vi "Write Roles.vi"(8 "error in (no error)":errorcluster, 10 "Roles":T1, 11 "PreparePassInGame1 in":refnum<class "PreparePassInGame1.lvclass">) -> (0 "error out":errorcluster, 3 "PreparePassInGame1 out":refnum<class "PreparePassInGame1.lvclass">)   [LabVIEW 2020, in "PreparePassInGame1.lvclass"]
uses:
  PreparePassInGame1.lvclass
  ShootRole_class/ShootRole.lvclass
  PreparePassReceiverRole_class/PreparePassReceiverRole.lvclass
  PreparePassInGame1.lvclass/PreparePassInGame1.ctl
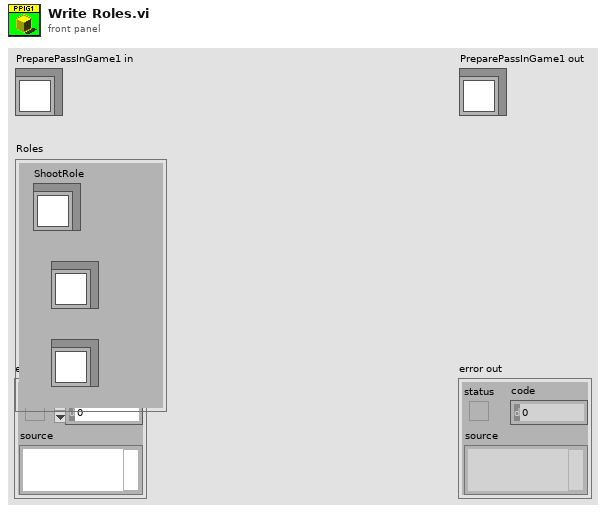
[diagram p1: front panel]
types:
  T1 = cluster{"ShootRole":refnum<class "ShootRole.lvclass">, "PreparePassReceiverRole1":refnum<class "PreparePassReceiverRole.lvclass">, "PreparePassReceiverRole2":refnum<class "PreparePassReceiverRole.lvclass">}
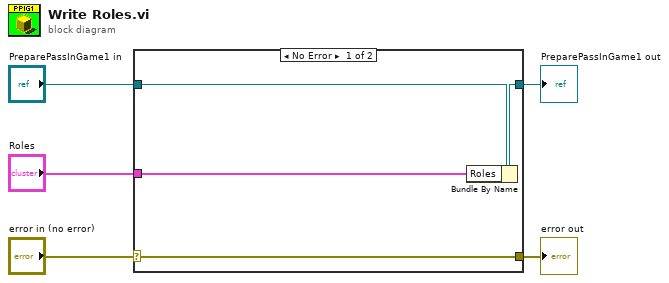
[diagram p0: block diagram]
diagram:
  n1 = case shown="No Error" "error in (no error)" {
    selector: "error in (no error)" -> [w9 w10]
    tunnel: [w9 w10] -> w4
    tunnel: [w7 w11] -> w2
    tunnel: "PreparePassInGame1 in" -> [w8 w11]
    tunnel: "Roles" -> [w6 _]
    frame No Error {
      n2 = Bundle By Name(cluster=w8, "Roles"=w6) -> (w7:refnum<class "PreparePassInGame1.lvclass">)
    }
    frame Error {
    }
  }
  "error out" <- w4
  "PreparePassInGame1 out" <- w2
